vi "诊断标定3 - 副本.vi"(8 "CAN端口":u16(ring), 9 "设备索引号":u16(ring), 10 "CAN卡类型":u32(ring)=21) -> ()   [LabVIEW 2013] (continued)
                                n3885 = local write "一级故障 2"(T10 {"总电压过高"=0.0, "整组电压不均衡"=0.0, "SOC过高"=0.0, "单体电压过高"=0.0, "总电压过低"=0.0, "温度过高"=0.0, "温度过低"=0.0, "单组电压不均衡"=0.0, "整组温度不均衡"=0.0, "单组温度不均衡"=0.0, "单体电压过低"=0.0, "充电电流过高"=0.0, "放电电流过高"=0.0, "SOC过低"=0.0, "内阻过大"=0.0, "极柱温度过高"=0.0, "SOH过低"=0.0} ("一级故障")) -> ()
                                }
                                frame "三级故障阀值" {
                                n3886 = local write "一级故障 3"(T10 {"总电压过高"=0.0, "整组电压不均衡"=0.0, "SOC过高"=0.0, "单体电压过高"=0.0, "总电压过低"=0.0, "温度过高"=0.0, "温度过低"=0.0, "单组电压不均衡"=0.0, "整组温度不均衡"=0.0, "单组温度不均衡"=0.0, "单体电压过低"=0.0, "充电电流过高"=0.0, "放电电流过高"=0.0, "SOC过低"=0.0, "内阻过大"=0.0, "极柱温度过高"=0.0, "SOH过低"=0.0} ("一级故障")) -> ()
                                }
                                frame "加热控制参数" {
                                n3887 = local write "加热控制参数"(T11 {"风机开启温度"=0.0, "风机关闭温度"=0.0, "加热开启温度"=0.0, "加热关闭温度"=0.0, "风机开启温差"=0.0, "风机关闭温差"=0.0, "加热关闭温差"=0.0} ("加热控制参数")) -> ()
                                }
                                frame "充电控制参数" {
                                n3888 = local write "一级故障 5"(T12 {"最大允许单体电压"=0.0, "最大允许总电压"=0.0, "最小允许单体电压"=0.0, "最大允许充电电流"=0.0, "最小允许充电电流"=0.0, "最大允许充电温度"=0.0, "最小允许充电温度"=0.0, "电流步长"=0.0} ("一级故障 5")) -> ()
                                }
                                frame "电池信息1" {
                                w5506 = ""
                                w5507 = 0.0 ("电池串联")
                                n3889 = local read "电池信息"() -> (w5509:T13)
                                n3890 = Bundle By Name(cluster=w5509, "电池串联"=w5507, "电池并联"=w5507, "电池包额定容量"=w5507, "电池包额定能量(kWh)"=w5507, "电池包额定总电压"=w5507, "实际容量"=w5507, "电池厂家"=w5506, "电池类型"=w5506, "电池生产日期"=w5506) -> (w5508:T13)
                                n3891 = local write "电池信息"(w5508) -> ()
                                }
                                frame "电池包组号" {
                                n3892 = local read "电池信息"() -> (w5512:T13)
                                n3893 = Bundle By Name(cluster=w5512, "电池包组号"="") -> (w5511:T13)
                                n3894 = local write "电池信息"(w5511) -> ()
                                }
                                frame "充放电安时" {
                                w5513 = 0.0 ("累计充电总安时")
                                n3895 = local read "电池信息"() -> (w5515:T13)
                                n3896 = Bundle By Name(cluster=w5515, "累计充电总安时"=w5513, "累计放电总安时"=w5513) -> (w5514:T13)
                                n3897 = local write "电池信息"(w5514) -> ()
                                }
                                frame "电池充放电次数" {
                                w5516 = 0.0 ("累计充电总安时")
                                n3898 = local read "电池信息"() -> (w5518:T13)
                                n3899 = Bundle By Name(cluster=w5518, "电池充满次数"=w5516, "电池放空次数"=w5516, "电池充电次数"=w5516) -> (w5517:T13)
                                n3900 = local write "电池信息"(w5517) -> ()
                                }
                                }
                              }
                              frame "从板" {
                                n3901 = case shown="\"温度起始值\"" w5519 {
                                frame "假", Default {
                                }
                                frame "电压起始值" {
                                n3902 = for {
                                N: 1 -> [_]
                                tunnel: [""] -> w5524 mode=indexing
                                }
                                n3903 = control-ref of="项目信息 2"() -> (w5520:refnum<vi>)
                                n3904 = call "表格数据输入-8.6.vi"("行数"=u32 0, "列数"=u32 1, "字符串数组"=w5524, "表格引用"=w5520) -> ()  [unwired: 8 in]
                                }
                                frame "通道电压个数" {
                                n3905 = for {
                                N: 5 -> [_]
                                tunnel: [""] -> w5530 mode=indexing
                                }
                                n3906 = control-ref of="项目信息 2"() -> (w5526:refnum<vi>)
                                n3907 = call "表格数据输入-8.6.vi"("行数"=u32 22, "列数"=u32 1, "字符串数组"=w5530, "表格引用"=w5526) -> ()  [unwired: 8 in]
                                }
                                frame "保险位置" {
                                n3908 = for {
                                N: 10 -> [_]
                                tunnel: [""] -> w5536 mode=indexing
                                }
                                n3909 = control-ref of="项目信息 2"() -> (w5532:refnum<vi>)
                                n3910 = call "表格数据输入-8.6.vi"("行数"=u32 2, "列数"=u32 1, "字符串数组"=w5536, "表格引用"=w5532) -> ()  [unwired: 8 in]
                                }
                                frame "温度起始值" {
                                n3911 = for {
                                N: 1 -> [_]
                                tunnel: [""] -> w5542 mode=indexing
                                }
                                n3912 = control-ref of="项目信息 2"() -> (w5538:refnum<vi>)
                                n3913 = call "表格数据输入-8.6.vi"("行数"=u32 1, "列数"=u32 1, "字符串数组"=w5542, "表格引用"=w5538) -> ()  [unwired: 8 in]
                                }
                                frame "加热控制参数" {
                                n3914 = local write "加热控制参数"(T11 {"风机开启温度"=0.0, "风机关闭温度"=0.0, "加热开启温度"=0.0, "加热关闭温度"=0.0, "风机开启温差"=0.0, "风机关闭温差"=0.0, "加热关闭温差"=0.0} ("加热控制参数")) -> ()
                                }
                                frame "一级故障阀值" {
                                n3915 = local write "一级故障 6"(T15 {"电压过高"=0.0, "电压过低"=0.0, "温度过高"=0.0, "温度过低"=0.0, "电压不均衡(V)"=0.0, "温度不均衡"=0.0, "SOC过低"=0.0} ("一级故障 6")) -> ()
                                }
                                frame "二级故障阀值" {
                                n3916 = local write "一级故障 7"(T15 {"电压过高"=0.0, "电压过低"=0.0, "温度过高"=0.0, "温度过低"=0.0, "电压不均衡(V)"=0.0, "温度不均衡"=0.0, "SOC过低"=0.0} ("一级故障 7")) -> ()
                                }
                                frame "三级故障阀值" {
                                n3917 = local write "一级故障 8"(T15 {"电压过高"=0.0, "电压过低"=0.0, "温度过高"=0.0, "温度过低"=0.0, "电压不均衡(V)"=0.0, "温度不均衡"=0.0, "SOC过低"=0.0} ("一级故障 7")) -> ()
                                }
                                frame "均衡参数" {
                                n3918 = local write "均衡参数"(T17 {"充电结束电压(90%)"=0.0, "充电结束电压(91%)"=0.0, "充电结束电压(92%)"=0.0, "充电结束电压(93%)"=0.0, "充电结束电压(94%)"=0.0, "均衡计算-电压高阀值1级"=0.0, "均衡计算-电压高阀值2级"=0.0, "均衡计算-电压低阀值1级"=0.0, "均衡计算-电压低阀值2级"=0.0, "均衡计算-最低电压阀值"=0.0, "均衡停止-最低电压阀值"=0.0, "均衡计算-电压极差阀值"=0.0, "充电结束电压(95%)"=0.0, "充电结束电压(96%)"=0.0, "充电结束电压(97%)"=0.0, "充电结束电压(98%)"=0.0, "充电结束电压(99%)"=0.0, "充电结束电压(100%)"=0.0} ("均衡参数")) -> ()
                                }
                                frame "均衡阀值" {
                                w5549 = sgl 0.0 ("均衡计算-电压高阀值1级")
                                n3919 = local read "均衡参数"() -> (w5550:T17)
                                n3920 = Bundle By Name(cluster=w5550, "均衡计算-电压高阀值1级"=w5549, "均衡计算-电压高阀值2级"=w5549, "均衡计算-电压低阀值1级"=w5549, "均衡计算-电压低阀值2级"=w5549, "均衡计算-最低电压阀值"=w5549, "均衡停止-最低电压阀值"=w5549, "均衡计算-电压极差阀值"=w5549) -> (w5551:T17)
                                n3921 = local write "均衡参数"(w5551) -> ()
                                }
                                frame "充电结束电压" {
                                w5552 = sgl 0.0 ("均衡计算-电压高阀值1级")
                                n3922 = local read "均衡参数"() -> (w5553:T17)
                                n3923 = Bundle By Name(cluster=w5553, "充电结束电压(90%)"=w5552, "充电结束电压(91%)"=w5552, "充电结束电压(92%)"=w5552, "充电结束电压(93%)"=w5552, "充电结束电压(94%)"=w5552, "充电结束电压(95%)"=w5552, "充电结束电压(96%)"=w5552, "充电结束电压(97%)"=w5552, "充电结束电压(98%)"=w5552, "充电结束电压(99%)"=w5552, "充电结束电压(100%)"=w5552) -> (w5554:T17)
                                n3924 = local write "均衡参数"(w5554) -> ()
                                }
                                }
                              }
                            }
                          }
                          frame #1 {
                            w5555 = FALSE ("流控帧")
                            w5556 = TRUE ("流控帧 2")
                            n3925 = global write "EV05全局变量1.vi" "写入超时"(w5555) -> ()
                            n3926 = global write "EV05全局变量1.vi" "流控帧"(w5555) -> ()
                            n3927 = local write "写?"(w5555) -> ()
                            n3928 = local write "消除"(w5556) -> ()
                            n3929 = local write "控制1"(w5556) -> ()
                            n3930 = global write "EV05全局变量1.vi" "流控帧 2"(w5556) -> ()
                          }
                          frame #2 {
                            n3931 = Wait Until Next ms Multiple(millisecond multiple=u32 300 ("毫秒倍数")) -> ()  [unwired: 1 out]
                          }
                          frame #3 {
                            n3932 = local read "设备索引号"() -> (w5559:u16)
                            n3933 = local read "CAN卡类型"() -> (w5560:u32)
                            n3934 = local read "CAN端口"() -> (w5558:u16)
                            n3935 = local write "命令序号"(w5563) -> ()
                            n3936 = stacked-sequence {
                              tunnel: w5564 -> [_ w5571]
                              tunnel: w5563 -> [_ w5570]
                              tunnel: w5562 -> [_ w5569]
                              tunnel: w5561 -> [_ w5568]
                              tunnel: w5560 -> [_ w5567]
                              tunnel: w5559 -> [_ w5566]
                              tunnel: w5558 -> [_ w5565]
                              frame #0 {
                              }
                              frame #1 {
                                n3937 = call "多帧发送机制(EV05).vi"("can卡类型"=w5567, "设备索引号"=w5566, "CAN端口"=w5565, "命令"=w5571, "板号"=w5569, "命令序号"=w5570, "输入数据"=w5568) -> ()  [unwired: 1 in, 12 out]
                              }
                            }
                          }
                          frame #4 {
                            n3938 = while {
                              tunnel: [w5576] -> w5573
                              tunnel: [w5575] -> w5572
                              i -> [w5579]
                              stop <- w5576 stop-if-true
                              n3939 = local read "强制终止读写标记"() -> (w5574:bool)
                              n3940 = global read "EV05全局变量1.vi" "写入超时"() -> (w5575:bool)
                              n3941 = Greater Or Equal?(x=w5579, y=20) -> (x >= y?=w5577:bool)
                              n3942 = Compound Arithmetic op=OR(w5574, w5575, w5577) -> (w5576:bool)
                              n3943 = Wait Until Next ms Multiple(millisecond multiple=u32 100 ("毫秒倍数")) -> ()  [unwired: 1 out]
                            }
                          }
                          frame #5 {
                            n3944 = case shown="假" w5588 {
                              tunnel: w5587 -> [w5599 _]
                              tunnel: [w5594 w5611] -> w5586
                              tunnel: w5585 -> [w5593 _]
                              tunnel: w5584 -> [w5592 w5611]
                              tunnel: [w5591 w5610] -> w5581
                              tunnel: w5583 -> [w5590 _]
                              tunnel: w5582 -> [w5589 w5610]
                              frame False {
                                n3945 = local read "重试次数"() -> (w5598:u8)
                                n3946 = Increment(x=w5598) -> (x+1=w5597:u8)
                                n3947 = local write "重试次数"(w5597) -> ()
                                n3948 = Greater Or Equal?(x=w5597, y=u8 4) -> (x >= y?=w5596:bool)
                                n3949 = case shown="真" w5596 {
                                tunnel: w5599 -> [_ w5604]
                                tunnel: [w5601 w5603] -> w5594
                                tunnel: w5593 -> [w5601 _]
                                tunnel: w5592 -> [_ w5603]
                                tunnel: [w5600 w5602] -> w5591
                                tunnel: w5590 -> [w5600 _]
                                tunnel: w5589 -> [_ w5602]
                                frame False {
                                }
                                frame True {
                                n3950 = control-ref of="结果"() -> (w5606:refnum<vi>)
                                n3951 = Concatenate Strings(w5604, "     读取失败" ("字符串")) -> (w5608:string)
                                n3952 = Build Array(w5608) -> (w5605:string[])
                                n3953 = call "表格编辑.vi"("新元素/子数组"=w5605, "活动单元格:单元格背景色"=u32 16740749, "MCListbox引用句柄"=w5606) -> ()  [unwired: 9 out]
                                }
                                }
                              }
                              frame True {
                              }
                            }
                          }
                          frame #6 {
                            n3954 = And(x=w5613, y=w5615) -> (x .and. y?=w5614:bool)
                            n3955 = case shown="真" w5614 {
                              frame False {
                              }
                              frame True {
                                n3956 = local write "强制终止读写标记"(FALSE ("强制停止")) -> ()
                                n3957 = control-ref of="结果"() -> (w5618:refnum<vi>)
                                n3958 = Concatenate Strings("读取完成" ("字符串")) -> (w5620:string)
                                n3959 = Build Array(w5620) -> (w5617:string[])
                                n3960 = call "表格编辑.vi"("新元素/子数组"=w5617, "活动单元格:单元格背景色"=u32 21937, "MCListbox引用句柄"=w5618) -> ()  [unwired: 9 out]
                              }
                            }
                            n3961 = Wait (ms)(milliseconds to wait=u32 50 ("等待时间（毫秒）")) -> ()  [unwired: 1 out]
                          }
                        }
                      }
                    }
                  }
                  n3962 = local read "强制终止读写标记"() -> (w5386:bool)
                  n3963 = Or(x=w5386, y=w5385) -> (x .or. y?=w5383:bool)
                }
              }
            }
            frame #2 {
              n3964 = case shown="假" w5705 {
                tunnel: w5706 -> [w5707 _]
                frame False {
                  n3965 = case shown="\"主板\", 默认" w5707 {
                    frame "主板", Default {
                      n3966 = global read "读配置文件全局.vi" "电池额定实际容量判定"() -> (w5721:bool)
                      n3967 = global read "读配置文件全局.vi" "电池充放电次数判定"() -> (w5710:bool)
                      n3968 = global read "读配置文件全局.vi" "加热控制参数判定"() -> (w5708:bool)
                      n3969 = global read "读配置文件全局.vi" "配置文件版本判定"() -> (w5720:bool)
                      n3970 = global read "读配置文件全局.vi" "充电控制参数判定"() -> (w5714:bool)
                      n3971 = global read "读配置文件全局.vi" "通道电压数判定"() -> (w5726:bool)
                      n3972 = global read "读配置文件全局.vi" "电压起始值判定"() -> (w5725:bool)
                      n3973 = global read "读配置文件全局.vi" "温度起始值判定"() -> (w5723:bool)
                      n3974 = global read "读配置文件全局.vi" "充放电安时判定"() -> (w5712:bool)
                      n3975 = global read "读配置文件全局.vi" "电池包组号判定"() -> (w5711:bool)
                      n3976 = global read "读配置文件全局.vi" "电池信息1判定"() -> (w5713:bool)
                      n3977 = global read "读配置文件全局.vi" "从板个数判定"() -> (w5729:bool)
                      n3978 = global read "读配置文件全局.vi" "产品编号判定"() -> (w5728:bool)
                      n3979 = global read "读配置文件全局.vi" "电压个数判定"() -> (w5727:bool)
                      n3980 = global read "读配置文件全局.vi" "温度个数判定"() -> (w5724:bool)
                      n3981 = global read "读配置文件全局.vi" "保险位置判定"() -> (w5722:bool)
                      n3982 = global read "读配置文件全局.vi" "一级故障判定"() -> (w5717:bool)
                      n3983 = global read "读配置文件全局.vi" "二级故障判定"() -> (w5716:bool)
                      n3984 = global read "读配置文件全局.vi" "三级故障判定"() -> (w5715:bool)
                      n3985 = global read "读配置文件全局.vi" "车牌号判定"() -> (w5719:bool)
                      n3986 = global read "读配置文件全局.vi" "SOH判定"() -> (w5718:bool)
                      n3987 = Build Array(w5729, w5728, w5727, w5726, w5725, w5724, w5723, w5722, w5721, w5720, w5719, w5718, w5717, w5716, w5715, w5714, w5713, w5712, w5711, w5710, w5708) -> (w5709:bool[])
                      n3988 = And Array Elements(Boolean array=w5709) -> (logical AND=w5730:bool)
                      n3989 = disable-structure shown="禁用" {
                        frame Disabled {
                          n3990 = global read "读配置文件全局.vi" "SOC判定"() -> ()  [unwired: 1 out]
                        }
                        frame Enabled {
                        }
                      }
                      n3991 = case shown="假" w5730 {
                        tunnel: w5709 -> [_ w5735]
                        frame True {
                          n3992 = control-ref of="结果"() -> (w5733:refnum<vi>)
                          n3993 = Build Array("全部判定成功!!!!!!!!") -> (w5734:string[])
                          n3994 = call "表格编辑.vi"("新元素/子数组"=w5734, "活动单元格:单元格背景色"=u32 6618880, "MCListbox引用句柄"=w5733) -> ()  [unwired: 9 out]
                        }
                        frame False {
                          n3995 = stacked-sequence {
                            tunnel: w5735 -> [_ w5740]
                            frame #0 {
                              n3996 = control-ref of="结果"() -> (w5738:refnum<vi>)
                              n3997 = Build Array("全部判定失败!!!!!") -> (w5739:string[])
                              n3998 = call "表格编辑.vi"("新元素/子数组"=w5739, "活动单元格:单元格背景色"=u32 16711680, "MCListbox引用句柄"=w5738) -> ()  [unwired: 9 out]
                            }
                            frame #1 {
                              n3999 = for {
                                tunnel: w5740 -> [w5742] mode=indexing
                                i -> [w5741]
                                n4000 = case shown="20" w5741 {
                                tunnel: w5742 -> [w5743 w5748 w5753 w5758 w5763 w5768 w5773 w5778 w5783 w5788 w5793 w5798 w5803 w5808 w5813 w5818 w5823 w5828 w5833 w5838 w5843 _]
                                frame 0 {
                                n4001 = case shown="假" w5743 {
                                frame False {
                                n4002 = control-ref of="结果"() -> (w5746:refnum<vi>)
                                n4003 = Build Array("从板个数判定失败!") -> (w5747:string[])
                                n4004 = call "表格编辑.vi"("新元素/子数组"=w5747, "活动单元格:单元格背景色"=u32 16711680, "MCListbox引用句柄"=w5746) -> ()  [unwired: 9 out]
                                }
                                frame True {
                                }
                                }
                                }
                                frame 1 {
                                n4005 = case shown="假" w5748 {
                                frame False {
                                n4006 = control-ref of="结果"() -> (w5751:refnum<vi>)
                                n4007 = Build Array("产品编号判定失败!") -> (w5752:string[])
                                n4008 = call "表格编辑.vi"("新元素/子数组"=w5752, "活动单元格:单元格背景色"=u32 16711680, "MCListbox引用句柄"=w5751) -> ()  [unwired: 9 out]
                                }
                                frame True {
                                }
                                }
                                }
                                frame 2 {
                                n4009 = case shown="假" w5753 {
                                frame False {
                                n4010 = control-ref of="结果"() -> (w5756:refnum<vi>)
                                n4011 = Build Array("电压个数判定失败!") -> (w5757:string[])
                                n4012 = call "表格编辑.vi"("新元素/子数组"=w5757, "活动单元格:单元格背景色"=u32 16711680, "MCListbox引用句柄"=w5756) -> ()  [unwired: 9 out]
                                }
                                frame True {
                                }
                                }
                                }
                                frame 3 {
                                n4013 = case shown="假" w5758 {
                                frame False {
                                n4014 = control-ref of="结果"() -> (w5761:refnum<vi>)
                                n4015 = Build Array("通道电压数判定失败!") -> (w5762:string[])
                                n4016 = call "表格编辑.vi"("新元素/子数组"=w5762, "活动单元格:单元格背景色"=u32 16711680, "MCListbox引用句柄"=w5761) -> ()  [unwired: 9 out]
                                }
                                frame True {
                                }
                                }
                                }
                                frame 4 {
                                n4017 = case shown="假" w5763 {
                                frame False {
                                n4018 = control-ref of="结果"() -> (w5766:refnum<vi>)
                                n4019 = Build Array("电压起始值判定失败!") -> (w5767:string[])
                                n4020 = call "表格编辑.vi"("新元素/子数组"=w5767, "活动单元格:单元格背景色"=u32 16711680, "MCListbox引用句柄"=w5766) -> ()  [unwired: 9 out]
                                }
                                frame True {
                                }
                                }
                                }
                                frame 5 {
                                n4021 = case shown="假" w5768 {
                                frame False {
                                n4022 = control-ref of="结果"() -> (w5771:refnum<vi>)
                                n4023 = Build Array("温度个数判定失败!") -> (w5772:string[])
                                n4024 = call "表格编辑.vi"("新元素/子数组"=w5772, "活动单元格:单元格背景色"=u32 16711680, "MCListbox引用句柄"=w5771) -> ()  [unwired: 9 out]
                                }
                                frame True {
                                }
                                }
                                }
                                frame 6 {
                                n4025 = case shown="假" w5773 {
                                frame False {
                                n4026 = control-ref of="结果"() -> (w5776:refnum<vi>)
                                n4027 = Build Array("温度起始值判定失败!") -> (w5777:string[])
                                n4028 = call "表格编辑.vi"("新元素/子数组"=w5777, "活动单元格:单元格背景色"=u32 16711680, "MCListbox引用句柄"=w5776) -> ()  [unwired: 9 out]
                                }
                                frame True {
                                }
                                }
                                }
                                frame 7 {
                                n4029 = case shown="假" w5778 {
                                frame False {
                                n4030 = control-ref of="结果"() -> (w5781:refnum<vi>)
                                n4031 = Build Array("保险位置判定失败!") -> (w5782:string[])
                                n4032 = call "表格编辑.vi"("新元素/子数组"=w5782, "活动单元格:单元格背景色"=u32 16711680, "MCListbox引用句柄"=w5781) -> ()  [unwired: 9 out]
                                }
                                frame True {
                                }
                                }
                                }
                                frame 8 {
                                n4033 = case shown="假" w5783 {
                                frame False {
                                n4034 = control-ref of="结果"() -> (w5786:refnum<vi>)
                                n4035 = Build Array("电池额定实际容量判定失败!") -> (w5787:string[])
                                n4036 = call "表格编辑.vi"("新元素/子数组"=w5787, "活动单元格:单元格背景色"=u32 16711680, "MCListbox引用句柄"=w5786) -> ()  [unwired: 9 out]
                                }
                                frame True {
                                }
                                }
                                }
                                frame 9 {
                                n4037 = case shown="假" w5788 {
                                frame False {
                                n4038 = control-ref of="结果"() -> (w5791:refnum<vi>)
                                n4039 = Build Array("配置文件版本判定失败!") -> (w5792:string[])
                                n4040 = call "表格编辑.vi"("新元素/子数组"=w5792, "活动单元格:单元格背景色"=u32 16711680, "MCListbox引用句柄"=w5791) -> ()  [unwired: 9 out]
                                }
                                frame True {
                                }
                                }
                                }
                                frame 10 {
                                n4041 = case shown="假" w5793 {
                                frame False {
                                n4042 = control-ref of="结果"() -> (w5796:refnum<vi>)
                                n4043 = Build Array("车牌号判定失败!") -> (w5797:string[])
                                n4044 = call "表格编辑.vi"("新元素/子数组"=w5797, "活动单元格:单元格背景色"=u32 16711680, "MCListbox引用句柄"=w5796) -> ()  [unwired: 9 out]
                                }
                                frame True {
                                }
                                }
                                }
                                frame 11 {
                                n4045 = case shown="假" w5798 {
                                frame False {
                                n4046 = control-ref of="结果"() -> (w5801:refnum<vi>)
                                n4047 = Build Array("SOH判定失败!") -> (w5802:string[])
                                n4048 = call "表格编辑.vi"("新元素/子数组"=w5802, "活动单元格:单元格背景色"=u32 16711680, "MCListbox引用句柄"=w5801) -> ()  [unwired: 9 out]
                                }
                                frame True {
                                }
                                }
                                }
                                frame 12 {
                                n4049 = case shown="假" w5803 {
                                frame False {
                                n4050 = control-ref of="结果"() -> (w5806:refnum<vi>)
                                n4051 = Build Array("一级故障阀值判定失败!") -> (w5807:string[])
                                n4052 = call "表格编辑.vi"("新元素/子数组"=w5807, "活动单元格:单元格背景色"=u32 16711680, "MCListbox引用句柄"=w5806) -> ()  [unwired: 9 out]
                                }
                                frame True {
                                }
                                }
                                }
                                frame 13 {
                                n4053 = case shown="假" w5808 {
                                frame False {
                                n4054 = control-ref of="结果"() -> (w5811:refnum<vi>)
                                n4055 = Build Array("二级故障阀值判定失败!") -> (w5812:string[])
                                n4056 = call "表格编辑.vi"("新元素/子数组"=w5812, "活动单元格:单元格背景色"=u32 16711680, "MCListbox引用句柄"=w5811) -> ()  [unwired: 9 out]
                                }
                                frame True {
                                }
                                }
                                }
                                frame 14 {
                                n4057 = case shown="假" w5813 {
                                frame False {
                                n4058 = control-ref of="结果"() -> (w5816:refnum<vi>)
                                n4059 = Build Array("三级故障阀值判定失败!") -> (w5817:string[])
                                n4060 = call "表格编辑.vi"("新元素/子数组"=w5817, "活动单元格:单元格背景色"=u32 16711680, "MCListbox引用句柄"=w5816) -> ()  [unwired: 9 out]
                                }
                                frame True {
                                }
                                }
                                }
                                frame 15 {
                                n4061 = case shown="假" w5818 {
                                frame False {
                                n4062 = control-ref of="结果"() -> (w5821:refnum<vi>)
                                n4063 = Build Array("充电控制参数判定失败!") -> (w5822:string[])
                                n4064 = call "表格编辑.vi"("新元素/子数组"=w5822, "活动单元格:单元格背景色"=u32 16711680, "MCListbox引用句柄"=w5821) -> ()  [unwired: 9 out]
                                }
                                frame True {
                                }
                                }
                                }
                                frame 16 {
                                n4065 = case shown="假" w5823 {
                                frame False {
                                n4066 = control-ref of="结果"() -> (w5826:refnum<vi>)
                                n4067 = Build Array("电池信息1判定失败!") -> (w5827:string[])
                                n4068 = call "表格编辑.vi"("新元素/子数组"=w5827, "活动单元格:单元格背景色"=u32 16711680, "MCListbox引用句柄"=w5826) -> ()  [unwired: 9 out]
                                }
                                frame True {
                                }
                                }
                                }
                                frame 17 {
                                n4069 = case shown="假" w5828 {
                                frame False {
                                n4070 = control-ref of="结果"() -> (w5831:refnum<vi>)
                                n4071 = Build Array("充放电安时判定失败!") -> (w5832:string[])
                                n4072 = call "表格编辑.vi"("新元素/子数组"=w5832, "活动单元格:单元格背景色"=u32 16711680, "MCListbox引用句柄"=w5831) -> ()  [unwired: 9 out]
                                }
                                frame True {
                                }
                                }
                                }
                                frame 18 {
                                n4073 = case shown="假" w5833 {
                                frame False {
                                n4074 = control-ref of="结果"() -> (w5836:refnum<vi>)
                                n4075 = Build Array("电池包组号判定失败!") -> (w5837:string[])
                                n4076 = call "表格编辑.vi"("新元素/子数组"=w5837, "活动单元格:单元格背景色"=u32 16711680, "MCListbox引用句柄"=w5836) -> ()  [unwired: 9 out]
                                }
                                frame True {
                                }
                                }
                                }
                                frame 19 {
                                n4077 = case shown="假" w5838 {
                                frame False {
                                n4078 = control-ref of="结果"() -> (w5841:refnum<vi>)
                                n4079 = Build Array("电池充放电次数判定失败!") -> (w5842:string[])
                                n4080 = call "表格编辑.vi"("新元素/子数组"=w5842, "活动单元格:单元格背景色"=u32 16711680, "MCListbox引用句柄"=w5841) -> ()  [unwired: 9 out]
                                }
                                frame True {
                                }
                                }
                                }
                                frame 20 {
                                n4081 = case shown="假" w5843 {
                                frame False {
                                n4082 = control-ref of="结果"() -> (w5846:refnum<vi>)
                                n4083 = Build Array("加热控制参数判定失败!") -> (w5847:string[])
                                n4084 = call "表格编辑.vi"("新元素/子数组"=w5847, "活动单元格:单元格背景色"=u32 16711680, "MCListbox引用句柄"=w5846) -> ()  [unwired: 9 out]
                                }
                                frame True {
                                }
                                }
                                }
                                frame 99, Default {
                                }
                                }
                              }
                            }
                          }
                        }
                      }
                    }
                    frame "从板" {
                      n4085 = global read "读配置文件全局2.vi" "电压起始值判定"() -> (w5856:bool)
                      n4086 = global read "读配置文件全局2.vi" "温度起始值判定"() -> (w5853:bool)
                      n4087 = global read "读配置文件全局2.vi" "加热控制参数判定"() -> (w5848:bool)
                      n4088 = global read "读配置文件全局2.vi" "通道电压判定"() -> (w5855:bool)
                      n4089 = global read "读配置文件全局2.vi" "保险位置判定"() -> (w5854:bool)
                      n4090 = global read "读配置文件全局2.vi" "一级故障判定"() -> (w5851:bool)
                      n4091 = global read "读配置文件全局2.vi" "二级故障判定"() -> (w5850:bool)
                      n4092 = global read "读配置文件全局2.vi" "三级故障判定"() -> (w5849:bool)
                      n4093 = global read "读配置文件全局2.vi" "从板号判定"() -> (w5857:bool)
                      n4094 = Build Array(w5857, w5856, w5855, w5854, w5853, w5851, w5850, w5849, w5848) -> (w5852:bool[])
                      n4095 = And Array Elements(Boolean array=w5852) -> (logical AND=w5858:bool)
                      n4096 = case shown="假" w5858 {
                        tunnel: w5852 -> [_ w5863]
                        frame True {
                          n4097 = control-ref of="结果"() -> (w5861:refnum<vi>)
                          n4098 = Build Array("读取判定成功!!!!!!!!") -> (w5862:string[])
                          n4099 = call "表格编辑.vi"("新元素/子数组"=w5862, "活动单元格:单元格背景色"=u32 6618880, "MCListbox引用句柄"=w5861) -> ()  [unwired: 9 out]
                        }
                        frame False {
                          n4100 = stacked-sequence {
                            tunnel: w5863 -> [_ w5868]
                            frame #0 {
                              n4101 = control-ref of="结果"() -> (w5866:refnum<vi>)
                              n4102 = Build Array("读取判定失败!!!!!") -> (w5867:string[])
                              n4103 = call "表格编辑.vi"("新元素/子数组"=w5867, "活动单元格:单元格背景色"=u32 16711680, "MCListbox引用句柄"=w5866) -> ()  [unwired: 9 out]
                            }
                            frame #1 {
                              n4104 = for {
                                tunnel: w5868 -> [w5869] mode=indexing
                                i -> [w5870]
                                n4105 = case shown="0" w5870 {
                                tunnel: w5869 -> [w5871 w5876 w5881 w5886 w5891 w5896 w5901 w5906 w5911 _]
                                frame 0 {
                                n4106 = case shown="假" w5871 {
                                frame False {
                                n4107 = control-ref of="结果"() -> (w5874:refnum<vi>)
                                n4108 = Build Array("从板号判定失败!") -> (w5875:string[])
                                n4109 = call "表格编辑.vi"("新元素/子数组"=w5875, "活动单元格:单元格背景色"=u32 16711680, "MCListbox引用句柄"=w5874) -> ()  [unwired: 9 out]
                                }
                                frame True {
                                }
                                }
                                }
                                frame 1 {
                                n4110 = case shown="假" w5876 {
                                frame False {
                                n4111 = control-ref of="结果"() -> (w5879:refnum<vi>)
                                n4112 = Build Array("电压起始值判定失败!") -> (w5880:string[])
                                n4113 = call "表格编辑.vi"("新元素/子数组"=w5880, "活动单元格:单元格背景色"=u32 16711680, "MCListbox引用句柄"=w5879) -> ()  [unwired: 9 out]
                                }
                                frame True {
                                }
                                }
                                }
                                frame 2 {
                                n4114 = case shown="假" w5881 {
                                frame False {
                                n4115 = control-ref of="结果"() -> (w5884:refnum<vi>)
                                n4116 = Build Array("通道电压节数判定失败!") -> (w5885:string[])
                                n4117 = call "表格编辑.vi"("新元素/子数组"=w5885, "活动单元格:单元格背景色"=u32 16711680, "MCListbox引用句柄"=w5884) -> ()  [unwired: 9 out]
                                }
                                frame True {
                                }
                                }
                                }
                                frame 3 {
                                n4118 = case shown="假" w5886 {
                                frame False {
                                n4119 = control-ref of="结果"() -> (w5889:refnum<vi>)
                                n4120 = Build Array("保险位置判定失败!") -> (w5890:string[])
                                n4121 = call "表格编辑.vi"("新元素/子数组"=w5890, "活动单元格:单元格背景色"=u32 16711680, "MCListbox引用句柄"=w5889) -> ()  [unwired: 9 out]
                                }
                                frame True {
                                }
                                }
                                }
                                frame 4 {
                                n4122 = case shown="假" w5891 {
                                frame False {
                                n4123 = control-ref of="结果"() -> (w5894:refnum<vi>)
                                n4124 = Build Array("温度起始值判定失败!") -> (w5895:string[])
                                n4125 = call "表格编辑.vi"("新元素/子数组"=w5895, "活动单元格:单元格背景色"=u32 16711680, "MCListbox引用句柄"=w5894) -> ()  [unwired: 9 out]
                                }
                                frame True {
                                }
                                }
                                }
                                frame 5 {
                                n4126 = case shown="假" w5896 {
                                frame False {
                                n4127 = control-ref of="结果"() -> (w5899:refnum<vi>)
                                n4128 = Build Array("一级故障判定失败!") -> (w5900:string[])
                                n4129 = call "表格编辑.vi"("新元素/子数组"=w5900, "活动单元格:单元格背景色"=u32 16711680, "MCListbox引用句柄"=w5899) -> ()  [unwired: 9 out]
                                }
                                frame True {
                                }
                                }
                                }
                                frame 6 {
                                n4130 = case shown="假" w5901 {
                                frame False {
                                n4131 = control-ref of="结果"() -> (w5904:refnum<vi>)
                                n4132 = Build Array("二级故障判定失败!") -> (w5905:string[])
                                n4133 = call "表格编辑.vi"("新元素/子数组"=w5905, "活动单元格:单元格背景色"=u32 16711680, "MCListbox引用句柄"=w5904) -> ()  [unwired: 9 out]
                                }
                                frame True {
                                }
                                }
                                }
                                frame 7 {
                                n4134 = case shown="假" w5906 {
                                frame False {
                                n4135 = control-ref of="结果"() -> (w5909:refnum<vi>)
                                n4136 = Build Array("三级故障判定失败!") -> (w5910:string[])
                                n4137 = call "表格编辑.vi"("新元素/子数组"=w5910, "活动单元格:单元格背景色"=u32 16711680, "MCListbox引用句柄"=w5909) -> ()  [unwired: 9 out]
                                }
                                frame True {
                                }
                                }
                                }
                                frame 8 {
                                n4138 = case shown="假" w5911 {
                                frame False {
                                n4139 = control-ref of="结果"() -> (w5914:refnum<vi>)
                                n4140 = Build Array("加热控制参数判定失败!") -> (w5915:string[])
                                n4141 = call "表格编辑.vi"("新元素/子数组"=w5915, "活动单元格:单元格背景色"=u32 16711680, "MCListbox引用句柄"=w5914) -> ()  [unwired: 9 out]
                                }
                                frame True {
                                }
                                }
                                }
                                frame 99, Default {
                                }
                                }
                              }
                            }
                          }
                        }
                      }
                      n4142 = disable-structure shown="禁用" {
                        frame Disabled {
                          n4143 = global read "读配置文件全局.vi" "SOC判定"() -> ()  [unwired: 1 out]
                        }
                        frame Enabled {
                        }
                      }
                    }
                  }
                }
                frame True {
                }
              }
            }
          }
          n4144 = stacked-sequence {
            tunnel: w5148 -> [_]
            frame #0 {
              n4145 = local write "强制终止读写标记"(FALSE ("强制停止")) -> ()
            }
          }
          "重试次数" <- u8 0 ("重试次数")
        }
        frame "开启均衡" {
          n4146 = local read "从板板号"() -> (w5916:u8)
          n4147 = stacked-sequence {
            tunnel: 133 -> [_ w5942 _ _]
            tunnel: w5916 -> [_ _ _ _]
            frame #0 {
              w5926 = u8 0 items=["Normal", "Listen Only"] ("工作方式")
              w5925 = u8 1 items=["Dual Filter", "Single Filter"] ("滤波方式")
              n4148 = global write "EV05全局变量1.vi" "读取超时"(FALSE ("读取超时")) -> ()
              n4149 = global write "EV05全局变量1.vi" "流控帧 2"(TRUE ("流控帧 2")) -> ()
              n4150 = local write "写?"(TRUE ("写?")) -> ()
              n4151 = local read "设备索引号"() -> (w5921:u16)
              n4152 = local read "CAN卡类型"() -> (w5920:u32)
              n4153 = local read "CAN端口"() -> (w5922:u16)
              n4154 = local write "控制1"(TRUE ("控制1")) -> ()
              n4155 = local write "消除"(TRUE ("消除")) -> ()
              n4156 = global write "EV05全局变量1.vi" "流控帧"(FALSE ("流控帧")) -> ()
              n4157 = call "CAN_Init-8.6.vi"("CAN卡类型"=w5920, "设备索引号"=w5921, "CAN端口"=w5922, "操作类型"=enum16{"初始化CAN", "关闭CAN"}."初始化CAN", "滤波方式"=w5925, "Accept Code"=u32 606601216, "簇"=T23 {"打开CAN"=FALSE, "初始化CAN"=TRUE, "开始CAN"=TRUE, "重启"=FALSE, "关闭CAN"=FALSE}, "Mask Code"=u32 524287 ("Accept Code"), "工作方式"=w5926, "是否滤波"=TRUE, "滤波选择"=T22 {"fiter_mode"=1, "fiter_endid"=75825152, "fiter_startid"=75890687}) -> ()  [unwired: 3 in, 6 out]
              n4158 = Wait Until Next ms Multiple(millisecond multiple=u32 20 ("毫秒倍数")) -> ()  [unwired: 1 out]
            }
            frame #1 {
              n4159 = local write "命令"(w5942) -> ()
              n4160 = call "ID组合.vi"("SA(4)"=0 ("PDU(1)"), "PS(3)"=63 ("PDU(1)"), "PF(2)"=w5942, "PDU(1)"=4) -> ("ID"=w5941:i32)  [unwired: 7 out]
              n4161 = local read "均衡类型选择"() -> (w5938:enum16{"放电均衡", "充电均衡", "充放电均衡"})
              n4162 = local read "设备索引号"() -> (w5947:u16)
              n4163 = local read "CAN卡类型"() -> (w5948:u32)
              n4164 = local read "CAN端口"() -> (w5946:u16)
              n4165 = local write "命令序号"(2) -> ()
              n4166 = Add(x=w5938, y=1) -> (x+y=w5936:i32)
              n4167 = Build Array(2, 2, w5936) -> (w5949:i32[])
              n4168 = call "transmit-8.6.vi"("can卡类型"=w5948, "设备索引号"=w5947, "CAN端口"=w5946, "ID"=w5941, "SendType"=u8 0, "Data"=w5949) -> ()  [unwired: 3 in, 11 out]
            }
            frame #2 {
              n4169 = Wait Until Next ms Multiple(millisecond multiple=u32 1000 ("毫秒倍数")) -> ()  [unwired: 1 out]
            }
            frame #3 {
              w5957 = u8 0 items=["Normal", "Listen Only"] ("工作方式")
              w5958 = u8 1 items=["Dual Filter", "Single Filter"] ("滤波方式")
              n4170 = global write "EV05全局变量1.vi" "流控帧 2"(FALSE ("流控帧 2")) -> ()
              n4171 = local read "CAN卡类型"() -> (w5963:u32)
              n4172 = local read "设备索引号"() -> (w5962:u16)
              n4173 = local read "CAN端口"() -> (w5961:u16)
              n4174 = local write "控制1"(FALSE ("控制1")) -> ()
              n4175 = local write "消除"(FALSE ("消除")) -> ()
              n4176 = call <vilib>:"Unset Busy.vi"() -> ()  [unwired: 2 in, 10 out]
              n4177 = call "CAN_Init-8.6.vi"("CAN卡类型"=w5963, "设备索引号"=w5962, "CAN端口"=w5961, "操作类型"=enum16{"初始化CAN", "关闭CAN"}."初始化CAN", "滤波方式"=w5958, "Accept Code"=u32 3221225472, "簇"=T23 {"打开CAN"=FALSE, "初始化CAN"=TRUE, "开始CAN"=TRUE, "重启"=FALSE, "关闭CAN"=FALSE}, "Mask Code"=u32 1073741823 ("Accept Code"), "工作方式"=w5957, "是否滤波"=TRUE, "滤波选择"=T22 {"fiter_mode"=1, "fiter_endid"=402653184, "fiter_startid"=419430399}) -> ()  [unwired: 3 in, 6 out]
            }
          }
        }
        frame "关闭均衡" {
          n4178 = local read "从板板号"() -> (w5967:u8)
          n4179 = stacked-sequence {
            tunnel: 133 -> [_ w5991 _ _]
            tunnel: w5967 -> [_ _ _ _]
            frame #0 {
              w5977 = u8 0 items=["Normal", "Listen Only"] ("工作方式")
              w5976 = u8 1 items=["Dual Filter", "Single Filter"] ("滤波方式")
              n4180 = global write "EV05全局变量1.vi" "读取超时"(FALSE ("读取超时")) -> ()
              n4181 = global write "EV05全局变量1.vi" "流控帧 2"(TRUE ("流控帧 2")) -> ()
              n4182 = local write "写?"(TRUE ("写?")) -> ()
              n4183 = local read "设备索引号"() -> (w5972:u16)
              n4184 = local read "CAN卡类型"() -> (w5971:u32)
              n4185 = local read "CAN端口"() -> (w5973:u16)
              n4186 = local write "控制1"(TRUE ("控制1")) -> ()
              n4187 = global write "EV05全局变量1.vi" "流控帧"(FALSE ("流控帧")) -> ()
              n4188 = local write "消除"(TRUE ("消除")) -> ()
              n4189 = call "CAN_Init-8.6.vi"("CAN卡类型"=w5971, "设备索引号"=w5972, "CAN端口"=w5973, "操作类型"=enum16{"初始化CAN", "关闭CAN"}."初始化CAN", "滤波方式"=w5976, "Accept Code"=u32 606601216, "簇"=T23 {"打开CAN"=FALSE, "初始化CAN"=TRUE, "开始CAN"=TRUE, "重启"=FALSE, "关闭CAN"=FALSE}, "Mask Code"=u32 524287 ("Accept Code"), "工作方式"=w5977, "是否滤波"=TRUE, "滤波选择"=T22 {"fiter_mode"=1, "fiter_endid"=75825152, "fiter_startid"=75890687}) -> ()  [unwired: 3 in, 6 out]
              n4190 = Wait Until Next ms Multiple(millisecond multiple=u32 20 ("毫秒倍数")) -> ()  [unwired: 1 out]
            }
            frame #1 {
              n4191 = local write "命令"(w5991) -> ()
              n4192 = call "ID组合.vi"("SA(4)"=0 ("PDU(1)"), "PS(3)"=63 ("PDU(1)"), "PF(2)"=w5991, "PDU(1)"=4) -> ("ID"=w5990:i32)  [unwired: 7 out]
              n4193 = local read "均衡类型选择"() -> (w6001:enum16{"放电均衡", "充电均衡", "充放电均衡"})
              n4194 = local write "命令序号"(3) -> ()
              n4195 = local read "设备索引号"() -> (w5996:u16)
              n4196 = local read "CAN卡类型"() -> (w5997:u32)
              n4197 = local read "CAN端口"() -> (w5995:u16)
              n4198 = Add(x=w6001, y=1) -> (x+y=w5999:i32)
              n4199 = Build Array(2, 3, w5999) -> (w5998:i32[])
              n4200 = call "transmit-8.6.vi"("can卡类型"=w5997, "设备索引号"=w5996, "CAN端口"=w5995, "ID"=w5990, "SendType"=u8 0, "Data"=w5998) -> ()  [unwired: 3 in, 11 out]
            }
            frame #2 {
              n4201 = Wait Until Next ms Multiple(millisecond multiple=u32 1000 ("毫秒倍数")) -> ()  [unwired: 1 out]
            }
            frame #3 {
              w6008 = u8 0 items=["Normal", "Listen Only"] ("工作方式")
              w6009 = u8 1 items=["Dual Filter", "Single Filter"] ("滤波方式")
              n4202 = local read "设备索引号"() -> (w6013:u16)
              n4203 = local read "CAN卡类型"() -> (w6014:u32)
              n4204 = global write "EV05全局变量1.vi" "流控帧 2"(FALSE ("流控帧 2")) -> ()
              n4205 = local read "CAN端口"() -> (w6012:u16)
              n4206 = local write "控制1"(FALSE ("控制1")) -> ()
              n4207 = local write "消除"(FALSE ("消除")) -> ()
              n4208 = call "CAN_Init-8.6.vi"("CAN卡类型"=w6014, "设备索引号"=w6013, "CAN端口"=w6012, "操作类型"=enum16{"初始化CAN", "关闭CAN"}."初始化CAN", "滤波方式"=w6009, "Accept Code"=u32 3221225472, "簇"=T23 {"打开CAN"=FALSE, "初始化CAN"=TRUE, "开始CAN"=TRUE, "重启"=FALSE, "关闭CAN"=FALSE}, "Mask Code"=u32 1073741823 ("Accept Code"), "工作方式"=w6008, "是否滤波"=TRUE, "滤波选择"=T22 {"fiter_mode"=1, "fiter_endid"=402653184, "fiter_startid"=419430399}) -> ()  [unwired: 3 in, 6 out]
              n4209 = call <vilib>:"Unset Busy.vi"() -> ()  [unwired: 2 in, 10 out]
            }
          }
        }
        frame "强制均衡" {
          n4210 = local read "从板板号"() -> (w6018:u8)
          n4211 = stacked-sequence {
            tunnel: 133 -> [_ w6049 _ _]
            tunnel: w6018 -> [_ _ _ _]
            frame #0 {
              w6028 = u8 0 items=["Normal", "Listen Only"] ("工作方式")
              w6027 = u8 1 items=["Dual Filter", "Single Filter"] ("滤波方式")
              n4212 = global write "EV05全局变量1.vi" "读取超时"(FALSE ("读取超时")) -> ()
              n4213 = global write "EV05全局变量1.vi" "流控帧 2"(TRUE ("流控帧 2")) -> ()
              n4214 = local write "写?"(TRUE ("写?")) -> ()
              n4215 = local read "设备索引号"() -> (w6023:u16)
              n4216 = local read "CAN卡类型"() -> (w6022:u32)
              n4217 = local write "控制1"(TRUE ("控制1")) -> ()
              n4218 = local read "CAN端口"() -> (w6024:u16)
              n4219 = local write "消除"(TRUE ("消除")) -> ()
              n4220 = global write "EV05全局变量1.vi" "流控帧"(FALSE ("流控帧")) -> ()
              n4221 = call "CAN_Init-8.6.vi"("CAN卡类型"=w6022, "设备索引号"=w6023, "CAN端口"=w6024, "操作类型"=enum16{"初始化CAN", "关闭CAN"}."初始化CAN", "滤波方式"=w6027, "Accept Code"=u32 606601216, "簇"=T23 {"打开CAN"=FALSE, "初始化CAN"=TRUE, "开始CAN"=TRUE, "重启"=FALSE, "关闭CAN"=FALSE}, "Mask Code"=u32 524287 ("Accept Code"), "工作方式"=w6028, "是否滤波"=TRUE, "滤波选择"=T22 {"fiter_mode"=1, "fiter_endid"=75825152, "fiter_startid"=75890687}) -> ()  [unwired: 3 in, 6 out]
              n4222 = Wait Until Next ms Multiple(millisecond multiple=u32 20 ("毫秒倍数")) -> ()  [unwired: 1 out]
            }
            frame #1 {
              n4223 = local read "强制类型"() -> (w6055:enum16{"全通道开启", "单通道开启", "清待均衡时间"})
              n4224 = case shown="\"清待均衡时间\"" w6055 {
                tunnel: [250 252 254] -> w6045
                tunnel: [_ w6074 _] -> w6044
                tunnel: [_ w6073 _] -> w6043
                tunnel: [_ w6064 _] -> w6042
                tunnel: [_ w6057 _] -> w6041
                frame "全通道开启", Default {
                }
                frame "单通道开启" {
                  n4225 = local read "均衡类型选择"() -> (w6072:enum16{"放电均衡", "充电均衡", "充放电均衡"})
                  n4226 = local read "均衡位置"() -> (w6067:u16)
                  n4227 = case shown="\"放电均衡\", 默认" w6072 {
                    tunnel: [0 1] -> w6071
                    frame "放电均衡", Default {
                    }
                    frame "充电均衡" {
                    }
                  }
                  n4228 = Multiply(x="均衡时间", y=6.0) -> (x*y=w6059:dbl)
                  n4229 = Quotient & Remainder(x=w6059, y=256.0) -> (x-y*floor(x/y)=w6057:dbl, floor(x/y)=w6058:dbl)
                  n4230 = call "二进制解析-8.6.vi"("索引"=1, "数值"=w6071) -> ("低位子数组"=w6062:i32[])  [unwired: 1 in, 2 out]
                  n4231 = Quotient & Remainder(x=w6067, y=256.0) -> (x-y*floor(x/y)=w6073:dbl, floor(x/y)=w6074:dbl)
                  n4232 = call "二进制解析-8.6.vi"("索引"=8, "数值"=w6058) -> ("低位子数组"=w6063:i32[])  [unwired: 1 in, 2 out]
                  n4233 = Replace Array Subset(array=w6063, new element=w6062, index=0 ("索引")) -> (w6060:i32[])
                  n4234 = call "数值二进制转十进制-8.6.vi"("子数组"=w6060) -> ("十进制数值"=w6064:i32)  [unwired: 4 in]
                }
                frame "清待均衡时间" {
                }
              }
              n4235 = local write "命令"(w6049) -> ()
              n4236 = call "ID组合.vi"("SA(4)"=0 ("PDU(1)"), "PS(3)"=63 ("PDU(1)"), "PF(2)"=w6049, "PDU(1)"=4) -> ("ID"=w6048:i32)  [unwired: 7 out]
              n4237 = local read "设备索引号"() -> (w6052:u16)
              n4238 = local read "CAN卡类型"() -> (w6053:u32)
              n4239 = local read "CAN端口"() -> (w6051:u16)
              n4240 = local write "命令序号"(w6045) -> ()
              n4241 = Build Array(6, 4, w6045, w6044, w6043, w6042, w6041) -> (w6054:dbl[])
              n4242 = call "transmit-8.6.vi"("can卡类型"=w6053, "设备索引号"=w6052, "CAN端口"=w6051, "ID"=w6048, "SendType"=u8 0, "Data"=w6054) -> ()  [unwired: 3 in, 11 out]
            }
            frame #2 {
              n4243 = Wait Until Next ms Multiple(millisecond multiple=u32 1000 ("毫秒倍数")) -> ()  [unwired: 1 out]
            }
            frame #3 {
              w6088 = u8 0 items=["Normal", "Listen Only"] ("工作方式")
              w6087 = u8 1 items=["Dual Filter", "Single Filter"] ("滤波方式")
              n4244 = global write "EV05全局变量1.vi" "流控帧 2"(FALSE ("流控帧 2")) -> ()
              n4245 = local write "控制1"(FALSE ("控制1")) -> ()
              n4246 = local read "设备索引号"() -> (w6083:u16)
              n4247 = local read "CAN卡类型"() -> (w6082:u32)
              n4248 = local write "消除"(FALSE ("消除")) -> ()
              n4249 = local read "CAN端口"() -> (w6084:u16)
              n4250 = call <vilib>:"Unset Busy.vi"() -> ()  [unwired: 2 in, 10 out]
              n4251 = call "CAN_Init-8.6.vi"("CAN卡类型"=w6082, "设备索引号"=w6083, "CAN端口"=w6084, "操作类型"=enum16{"初始化CAN", "关闭CAN"}."初始化CAN", "滤波方式"=w6087, "Accept Code"=u32 3221225472, "簇"=T23 {"打开CAN"=FALSE, "初始化CAN"=TRUE, "开始CAN"=TRUE, "重启"=FALSE, "关闭CAN"=FALSE}, "Mask Code"=u32 1073741823 ("Accept Code"), "工作方式"=w6088, "是否滤波"=TRUE, "滤波选择"=T22 {"fiter_mode"=1, "fiter_endid"=402653184, "fiter_startid"=419430399}) -> ()  [unwired: 3 in, 6 out]
            }
          }
        }
        frame "项目软件版本读取" {
          n4252 = stacked-sequence {
            seq-local: [_ w6109 _] -> [_ _ w6116]
            frame #0 {
              n4253 = local read "设备索引号"() -> (w6096:u16)
              n4254 = local read "CAN卡类型"() -> (w6097:u32)
              n4255 = local read "CAN端口"() -> (w6095:u16)
              n4256 = stacked-sequence {
                tunnel: w6097 -> [w6100 w6108]
                tunnel: w6096 -> [w6099 w6107]
                tunnel: w6095 -> [w6098 w6106]
                frame #0 {
                  n4257 = dll-call lib="PTH1mabs FBluewave New EnergySVN_WorkBMS_Monitor_Bnet01trunk参数设置data\nkerneldlls\nusbcan.dll" fn="VCI_ClearBuffer"("DeviceType"=w6100, "DeviceInd"=w6099, "CANInd"=w6098) -> (error out=w6101:errorcluster)  [unwired: 4 in, 4 out]
                  n4258 = call <vilib>:"Clear Errors.vi"("error in (no error)"=w6101) -> ()  [unwired: 6 in, 1 out]
                }
                frame #1 {
                  w6105 = u8 137 ("命令")
                  w6104 = u32 1 ("命令序号")
                  n4259 = local read "从板板号"() -> (w6102:u8)
                  n4260 = local write "命令"(w6105) -> ()
